vi "String Array to Path Array.vi"(1 "Array in":string[](array[string])) -> (0 "Array out":path[](array[path]))   [LabVIEW 2018]
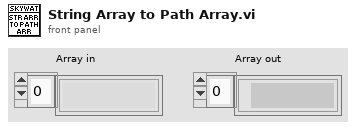
[diagram p1: front panel]
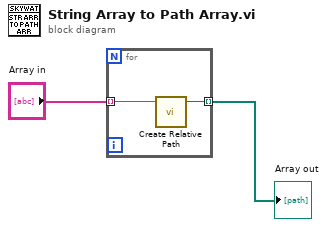
[diagram p0: block diagram]
diagram:
  n1 = for {
    tunnel: "Array in" -> [w4] mode=indexing
    tunnel: [w3] -> w2 mode=indexing
    n2 = call "Create Relative Path.vi"("file name"=w4) -> ("appended path"=w3:path)  [unwired: 4 in]
  }
  "Array out" <- w2
